vi "parse.vi"(8 "error in (no error)":errorcluster, 10 "DynamicFrameParser":refnum<class "DynamicFrameParser.lvclass">, 11 "HPILC in":refnum<class "HPILC.lvclass">) -> (0 "error out":errorcluster, 2 "ParseSuccessful":bool, 3 "HPILC out":refnum<class "HPILC.lvclass">)   [LabVIEW 2016, in "RTHPILC.lvlib" / "HPILC.lvclass"]
uses:
  HPILC.lvclass
  Common_RT_Modbus/DynamicFrameParser/DynamicFrameParser.lvclass
  Common_RT_ILC/ILC/ILC.lvclass
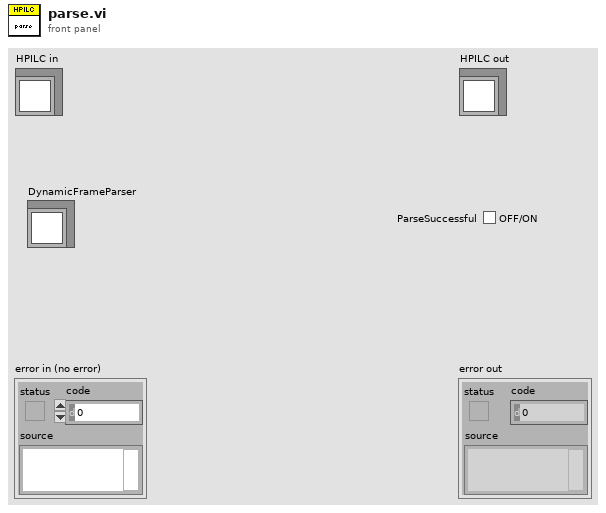
[diagram p1: front panel]
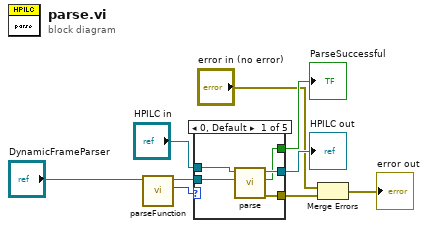
[diagram p0: block diagram]
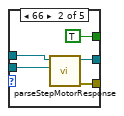
[diagram p2: hidden frame]
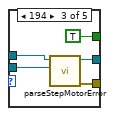
[diagram p3: hidden frame]
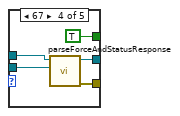
[diagram p4: hidden frame]
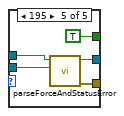
[diagram p5: hidden frame]
diagram:
  n1 = call "parseFunction.vi"("FrameParser in"="DynamicFrameParser") -> ("Function"=w8:u8, "FrameParser out"=w7:refnum<class "DynamicFrameParser.lvclass">)  [unwired: 8 in, 1 out]
  n2 = case shown="0, Default" w8 {
    tunnel: w7 -> [w14 w19 w23 w28 w33]
    tunnel: "HPILC in" -> [w13 w18 w24 w29 w34]
    tunnel: [w12 w17 w22 w25 w31] -> w5
    tunnel: [w11 TRUE ("ParseSuccessful") TRUE ("ParseSuccessful") TRUE ("ParseSuccessful") TRUE ("ParseSuccessful")] -> w4
    tunnel: [w10 w16 w20 w27 w32] -> w3
    frame 0, Default {
      n3 = call-parent "parse.vi"("DynamicFrameParser"=w14, "ILC in"=w13) -> ("error out"=w10:errorcluster, "ParseSuccessful"=w11:bool, "ILC out"=w12:refnum<class "HPILC.lvclass">)  [unwired: 7 in]
    }
    frame 66 {
      n4 = call "parseStepMotorResponse.vi"("DynamicFrameParser"=w19, "HPILC in"=w18) -> ("error out"=w16:errorcluster, "HPILC out"=w17:refnum<class "HPILC.lvclass">)  [unwired: 8 in]
    }
    frame 194 {
      n5 = call "parseStepMotorError.vi"("DynamicFrameParser"=w23, "HPILC in"=w24) -> ("error out"=w20:errorcluster, "HPILC out"=w22:refnum<class "HPILC.lvclass">)  [unwired: 8 in]
    }
    frame 67 {
      n6 = call "parseForceAndStatusResponse.vi"("DynamicFrameParser"=w28, "HPILC in"=w29) -> ("error out"=w27:errorcluster, "HPILC out"=w25:refnum<class "HPILC.lvclass">)  [unwired: 8 in]
    }
    frame 195 {
      n7 = call "parseForceAndStatusError.vi"("DynamicFrameParser"=w33, "HPILC in"=w34) -> ("error out"=w32:errorcluster, "HPILC out"=w31:refnum<class "HPILC.lvclass">)  [unwired: 8 in]
    }
  }
  "HPILC out" <- w5
  "ParseSuccessful" <- w4
  n8 = Merge Errors("error in (no error)", w3) -> (→"error out":errorcluster)
